vi "ScaleParamData1Pt.vi"(1 "max scale value":i16, 2 "parameter":u16(ring) items=["midband", "slope", "intercept"], 3 "Range Params":T1={"mb max"=-10.0, "mb min"=-60.0, "slope max"=4.0, "slope min"=-8.0, "int max"=5.0, "int min"=-85.0} {"int min" format="%.2f"; "int max" format="%.2f"; "slope min" format="%.2f"; "slope max" format="%.2f"; "mb min" format="%.2f"; "mb max" format="%.2f"}, 4 "raw image data in":dbl) -> (0 "scaled output":dbl)   [LabVIEW 2022 SP3]
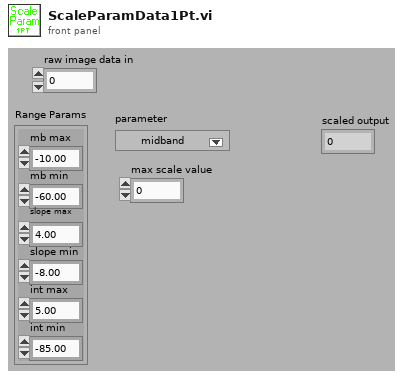
[diagram p1: front panel]
types:
  T1 = cluster{"mb max":dbl, "mb min":dbl, "slope max":dbl, "slope min":dbl, "int max":dbl, "int min":dbl}
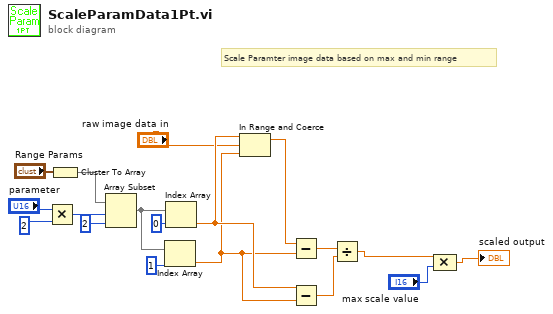
[diagram p0: block diagram]
diagram:
  # "Scale Paramter image data based on max and min range"
  n1 = Multiply(x="parameter", y=2) -> (x*y=w15:i32)
  n2 = Cluster To Array(cluster="Range Params") -> (array=w16:dbl[])
  n3 = Array Subset(array=w16, index=w15, length=2) -> (w12:dbl[])
  n4 = Index Array(array=w12, index=1) -> (element=w3:dbl)
  n5 = Index Array(array=w12, index=0) -> (element=w4:dbl)
  n6 = In Range and Coerce(upper limit=w4, x="raw image data in", lower limit=w3) -> (coerced(x)=w1:dbl)  [unwired: 1 out]
  n7 = Subtract(x=w1, y=w3) -> (x-y=w8:dbl)
  n8 = Subtract(x=w4, y=w3) -> (x-y=w7:dbl)
  n9 = Divide(x=w8, y=w7) -> (x/y=w5:dbl)
  n10 = Compound Arithmetic op=MULTIPLY(w5, "max scale value") -> (→"scaled output":dbl)
